vi "Pixmap laden.vi"(8 "error in (no error)":errorcluster caption="Fehler (Eingang, kein Fehler)", 11 "TDMS-Datei":refnum<k34>) -> (0 "error out":errorcluster caption="Fehler (Ausgang)", 2 "Pixmap":u32[][](array[numeric]), 3 "TDMS-Datei (Ausgang)":refnum<k34>)   [LabVIEW 2020, in "Anlagenuebersicht.lvlib" / "VisBx Anzeige.lvlib" / "TDMS laden.lvlib"]
doc: "Liest aus einer bereits geöffneten TDMS-Datei eine fertige Pixmap für die Darstellung eines Fixbildes."
uses:
  TDMS laden.lvlib
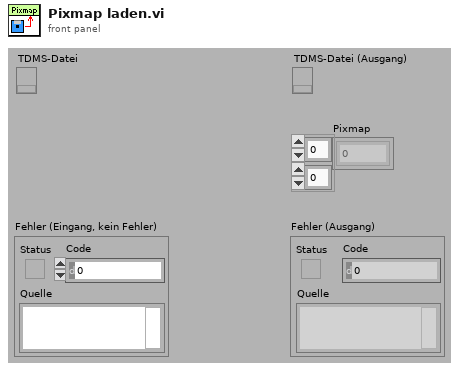
[diagram p1: front panel]
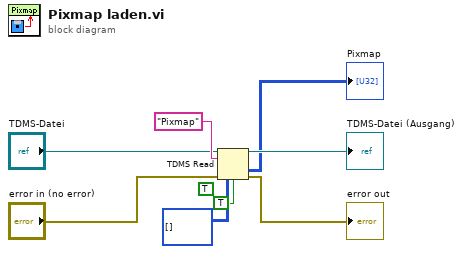
[diagram p0: block diagram]
diagram:
  (unwired) TRUE ("Kanalreihenfolge von Datei beibehalten? (F)")
  n1 = TDMS Read(0:"TDMS-Datei", 5:"Pixmap" ("Gruppenname (Eingang, Unbenannt)"), 11:"error in (no error)", 12:u32[][] [] ("Vorzeichenloses Byte-Array"), 13:TRUE ("Kanalreihenfolge von Datei beibehalten? (F)")) -> (4:→"TDMS-Datei (Ausgang)":refnum<k34>, 10:→"Pixmap":u32[][], 15:→"error out":errorcluster)  [unwired: 3 in, 3 out]
